vi "Read Data.vi"(8 "error in (no error)":errorcluster, 11 "EGG7260 in":refnum<class "EGG7260.lvclass">) -> (0 "error out":errorcluster, 2 "Data":waveform(dbl)[](array[waveform]), 3 "EGG7260 out":refnum<class "EGG7260.lvclass">)   [LabVIEW 2015, in "EGG7260.lvclass"]
uses:
  EGG7260.lvclass
  Instrument/Instrument.lvclass
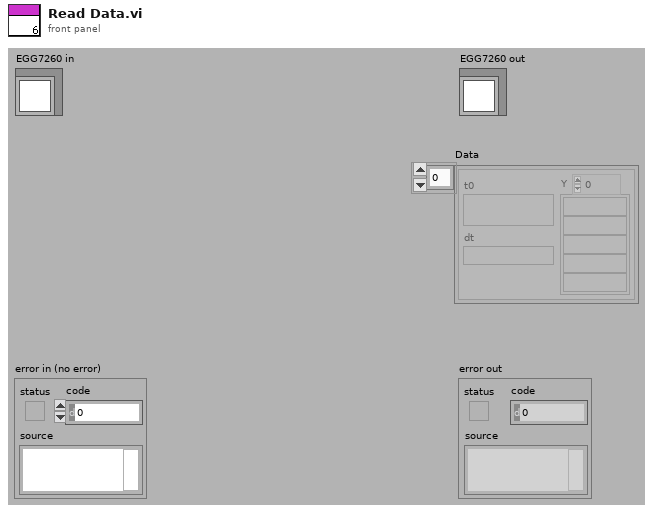
[diagram p1: front panel]
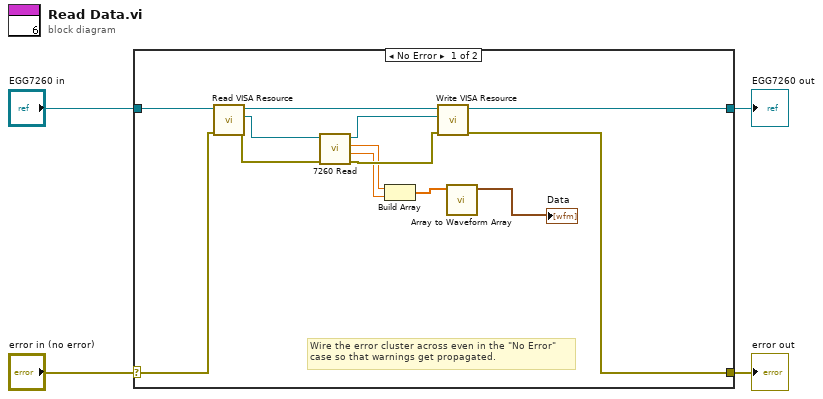
[diagram p0: block diagram]
diagram:
  n1 = case shown="No Error" "error in (no error)" {
    selector: "error in (no error)" -> [w12 w19]
    tunnel: [w9 w19] -> w3
    tunnel: [w15 w18] -> w1
    tunnel: "EGG7260 in" -> [w17 w18]
    frame No Error {
      # "Wire the error cluster across even in the \"No Error\"\ncase so that warnings get propagated."
      n2 = call "Read VISA Resource.vi"("error in (no error)"=w12, "Instrument.lvclass in"=w17) -> ("error out"=w11:errorcluster, "VISA Resource"=w14:refnum<visa-resource-name>, "Instrument.lvclass out"=w16:refnum<class "EGG7260.lvclass">)  [unwired: 7 out]
      n3 = call "7260 Read.vi"("error in (no error)"=w11, "VISA Resource Name"=w14) -> ("error out"=w10:errorcluster, "Y"=w6:dbl, "X"=w7:dbl, "VISA Resource Name Out"=w13:refnum<visa-resource-name>)  [unwired: 6 out]
      n4 = Build Array(w7, w6) -> (w8:dbl[])
      n5 = call "Write VISA Resource.vi"("error in (no error)"=w10, "VISA Resource"=w13, "Instrument.lvclass in"=w16) -> ("error out"=w9:errorcluster, "Instrument.lvclass out"=w15:refnum<class "EGG7260.lvclass">)  [unwired: 7 out]
      n6 = call "Array to Waveform Array.vi"("Array"=w8) -> ("Waveform"=→"Data":waveform(dbl)[])  [unwired: 10 in]
    }
    frame Error {
    }
  }
  "error out" <- w3
  "EGG7260 out" <- w1
